vi "SW_Fire_TTL_during_the_acquisition_universal.vi"(7 "IO inversion config.":u16, 8 "error in (no error)":errorcluster, 9 "Serial Port In":refnum<visa-resource-name>="COM3", 10 "TTL port(s) config to fire":u8, 11 "Fire TTL":bool) -> (0 "error out":errorcluster)   [LabVIEW 2018]
doc: "Fires TTL High to the TTL2 output for ~250 ms (default)."
panel:
  out "TTL has been reset":bool=TRUE
  out "TTL is fired":bool
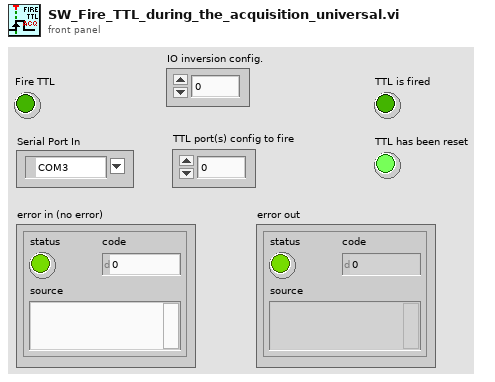
[diagram p1: front panel]
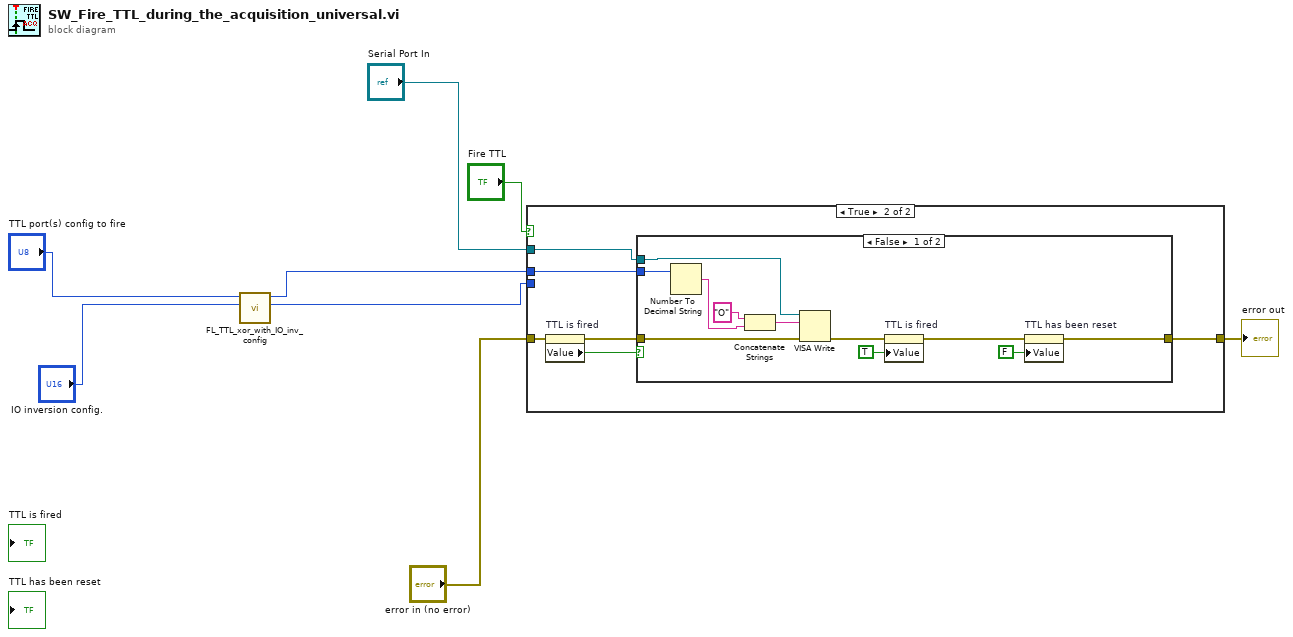
[diagram p0: block diagram]
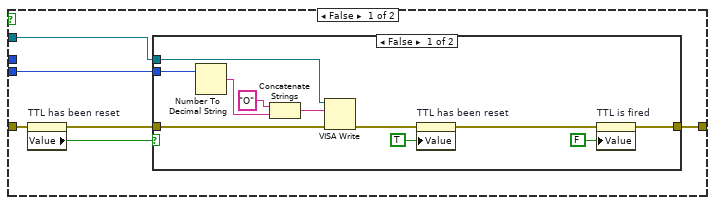
[diagram p2: hidden frame]
diagram:
  n1 = call "FL_TTL_xor_with_IO_inv_config.vi"("IO inversion config."="IO inversion config.", "TTL port(s) config to fire"="TTL port(s) config to fire") -> ("OFF config."=w1:u32, "ON config."=w2:u32)  [unwired: 8 in]
  n2 = case shown="True" "Fire TTL" {
    tunnel: "Serial Port In" -> [w14 w32]
    tunnel: "error in (no error)" -> [w13 w30]
    tunnel: [w11 w31] -> w6
    tunnel: w2 -> [_ w27]
    tunnel: w1 -> [w9 _]
    frame False {
      n3 = property on="TTL has been reset" class="Bool (strict)"(error in=w13) -> (error out=w12:errorcluster, "Value"=w10:bool)  [unwired: 1 in, 1 out]
      n4 = case shown="False" w10 {
        tunnel: w12 -> [w25 w26]
        tunnel: [w19 w26] -> w11
        tunnel: w14 -> [w24 _]
        tunnel: w9 -> [w15 _]
        frame False {
          n5 = Number To Decimal String(number=w15) -> (decimal integer string=w18:string)  [unwired: 1 in]
          n6 = Concatenate Strings("O" ("string"), w18) -> (w16:string)
          n7 = VISA Write(VISA resource name=w24, write buffer=w16, error in (no error)=w25) -> (error out=w23:errorcluster)  [unwired: 2 out]
          n8 = property on="TTL has been reset" class="Bool (strict)"(error in=w23, "Value"=TRUE ("TTL has been reset")) -> (error out=w20:errorcluster)  [unwired: 1 in, 1 out]
          n9 = property on="TTL is fired" class="Bool (strict)"(error in=w20, "Value"=FALSE ("TTL is fired")) -> (error out=w19:errorcluster)  [unwired: 1 in, 1 out]
        }
        frame True {
        }
      }
    }
    frame True {
      n10 = property on="TTL is fired" class="Bool (strict)"(error in=w30) -> (error out=w29:errorcluster, "Value"=w28:bool)  [unwired: 1 in, 1 out]
      n11 = case shown="False" w28 {
        tunnel: w32 -> [w39 _]
        tunnel: w29 -> [w38 w44]
        tunnel: [w40 w44] -> w31
        tunnel: w27 -> [w33 _]
        frame False {
          n12 = Number To Decimal String(number=w33) -> (decimal integer string=w35:string)  [unwired: 1 in]
          n13 = Concatenate Strings("O" ("string"), w35) -> (w36:string)
          n14 = VISA Write(VISA resource name=w39, write buffer=w36, error in (no error)=w38) -> (error out=w37:errorcluster)  [unwired: 2 out]
          n15 = property on="TTL is fired" class="Bool (strict)"(error in=w37, "Value"=TRUE ("TTL is fired")) -> (error out=w42:errorcluster)  [unwired: 1 in, 1 out]
          n16 = property on="TTL has been reset" class="Bool (strict)"(error in=w42, "Value"=FALSE ("TTL has been reset")) -> (error out=w40:errorcluster)  [unwired: 1 in, 1 out]
        }
        frame True {
        }
      }
    }
  }
  "error out" <- w6
